vi "plot data.vi"(0 "X":dbl, 1 "Boolean":bool, 5 "Y":dbl, 9 "Z":dbl) -> (4 "plots out":refnum<class "Base Datatype.lvclass">[](array[class]), 12 "arrayX":dbl[](array[numeric]), 13 "arrayY":dbl[](array[numeric]), 14 "arrayZ":dbl[](array[numeric]))   [LabVIEW 2014, in "HPCNC.lvlib"]
uses:
  <vilib>/Native 3D Graph/classes/Base Datatype.lvclass
  HPCNC.lvlib
  <vilib>/Native 3D Graph/xcontrol/3DPC_SurfacePlot.xctl
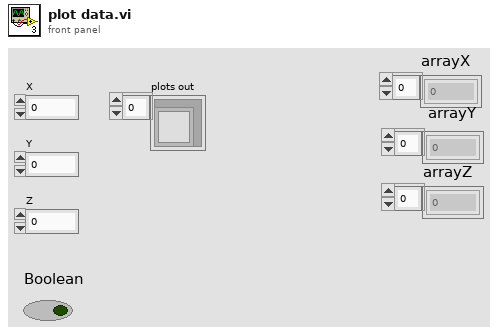
[diagram p1: front panel]
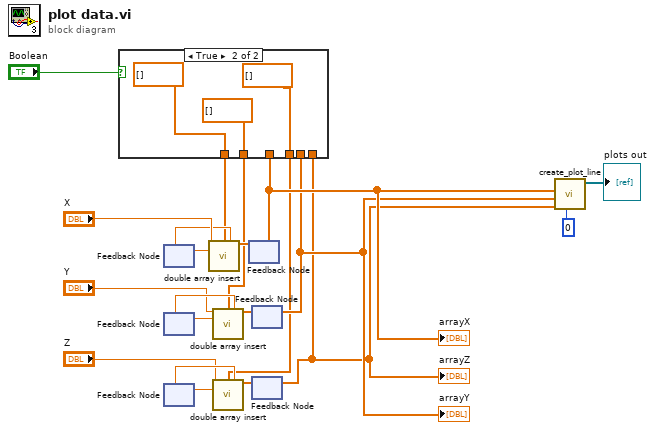
[diagram p0: block diagram]
diagram:
  n1 = feedback #1() -> (w17:dbl)  [unwired: 1 in]
  n2 = feedback #2() -> (w15:dbl)  [unwired: 1 in]
  n3 = feedback #3() -> (w11:dbl)  [unwired: 1 in]
  n4 = feedback #4() -> (w5:dbl[])  [unwired: 1 in]
  "arrayX" <- w5
  n5 = feedback #5() -> (w3:dbl[])  [unwired: 1 in]
  "arrayY" <- w3
  n6 = feedback #6() -> (w1:dbl[])  [unwired: 1 in]
  "arrayZ" <- w1
  n7 = case shown="True" "Boolean" {
    tunnel: [w24 dbl[] [] ("array")] -> w7
    tunnel: w5 -> [w24 _]
    tunnel: [w23 dbl[] [] ("array")] -> w4
    tunnel: w3 -> [w23 _]
    tunnel: [w22 dbl[] [] ("array")] -> w2
    tunnel: w1 -> [w22 _]
    frame False {
    }
    frame True {
    }
  }
  n8 = call "double array insert.vi"("Element"="X", "Array in"=w7, "Index"=w17) -> ("Array size"=w18:dbl, "Array out"=w6:dbl[])  [unwired: 11 in]
  n9 = feedback-in #1(w18) -> ()
  n10 = call "double array insert.vi"("Element"="Y", "Array in"=w4, "Index"=w15) -> ("Array size"=w16:dbl, "Array out"=w14:dbl[])  [unwired: 11 in]
  n11 = feedback-in #2(w16) -> ()
  n12 = call "double array insert.vi"("Element"="Z", "Array in"=w2, "Index"=w11) -> ("Array size"=w12:dbl, "Array out"=w10:dbl[])  [unwired: 11 in]
  n13 = feedback-in #3(w12) -> ()
  n14 = feedback-in #4(w6) -> ()
  n15 = feedback-in #5(w14) -> ()
  n16 = feedback-in #6(w10) -> ()
  n17 = call <vilib>:"create_plot_line.vi"("plot ID"=0, "z vector"=w1, "y vector"=w3, "x vector"=w5) -> ("plots out"=→"plots out":refnum<class "Base Datatype.lvclass">[])  [unwired: 2 in, 5 out]
